vi "MEMR-Initialize SGDA.vi"(0 "Data folder":path, 5 "Params":T32, 11 "error in (no error)":errorcluster) -> (4 "AO":T2 {"noiseChan"."Filter"."Stages"."IIR Filter"."Forward Coefficients" format="%.4f"; "noiseChan"."Filter"."Stages"."IIR Filter"."Reverse Coefficients" format="%.4f"}, 12 "Step In":T1, 14 "Step Out":T1, 15 "error out":errorcluster)   [LabVIEW 2020]
uses:
  Typedefs/MEMR-Params.ctl
  Typedefs/MEMR-Probe.ctl
  Typedefs/MEMR-Elicitor.ctl
  Human Studies/SFM Frontend/LV Source/Typedefs/HSTS-Transducer.ctl
  Typedefs/MEMR-Sequence.ctl
  Typedefs/MEMR-Analysis.ctl
  Typedefs/MEMR-Timing.ctl
  Typedefs/MEMR-AO Data.ctl
  Signal Synthesis VIs/3rd Generation/XControls/Stimulus Channel (G3)/Full Stimulus Channel Data.ctl
  Signal Synthesis VIs/3rd Generation/XControls/Waveform XControls/Waveform (G3)/Waveform Data.ctl
  Signal Synthesis VIs/3rd Generation/Waveform VIs/Waveform Enum (V3).ctl
  Signal Synthesis VIs/3rd Generation/XControls/Waveform XControls/Tone (G3)/Tone.Properties.ctl
  Signal Synthesis VIs/Waveform VIs/Pulse Train VIs/Pulse Train Params.ctl
  Signal Synthesis VIs/Waveform VIs/Pulse Train VIs/Pulse Polarity.ctl
  Signal Synthesis VIs/Waveform VIs/Pulse Train VIs/PT-Continuous State.ctl
  Signal Synthesis VIs/3rd Generation/Waveform VIs/Noise VIs/Noise (G3).ctl
  Signal Synthesis VIs/3rd Generation/Waveform VIs/Noise VIs/Noise (G3).Properties.ctl
  Signal Synthesis VIs/3rd Generation/Waveform VIs/Noise VIs/Noise (G3).Data.ctl
  Signal Synthesis VIs/Waveform VIs/File VIs/StimFile-Params.ctl
  Signal Synthesis VIs/Waveform VIs/FM Sweep VIs/FM Sweep Params.ctl
  Signal Synthesis VIs/Waveform VIs/Chirp Train VIs/Chirp Train.ctl
  Signal Synthesis VIs/Waveform VIs/Chirp Train VIs/Chirp Train Params.ctl
  Signal Synthesis VIs/Waveform VIs/Complex Tone VIs/CT-Params.ctl
  Signal Synthesis VIs/Waveform VIs/Complex Tone VIs/CT-Phase Enum.ctl
  Signal Synthesis VIs/Waveform VIs/Complex Tone VIs/CT-Runtime Data.ctl
  Signal Synthesis VIs/3rd Generation/XControls/Waveform XControls/FM Tone/Data.ctl
  Signal Synthesis VIs/3rd Generation/XControls/Waveform XControls/Vowel/Vowel.Properties.ctl
  Signal Synthesis VIs/3rd Generation/Waveform VIs/Ramp VIs/Ramp.Properties.ctl
  Signal Synthesis VIs/3rd Generation/XControls/Filter (G3)/Filter Data.ctl
  Signal Synthesis VIs/3rd Generation/XControls/Filter (G3)/Filter Type.ctl
  Signal Synthesis VIs/Filter VIs/Filter-Bandwidth Units.ctl
  Signal Synthesis VIs/Controls/Burst XCtl/Burst Data.ctl
  Signal Synthesis VIs/3rd Generation/XControls/Level (G3)/Level Data.ctl
  Signal Synthesis VIs/3rd Generation/XControls/Level (G3)/Level Units (G3).ctl
  Signal Synthesis VIs/3rd Generation/XControls/Advanced Options (G3)/Advanced Options (G3).ctl
  Signal Synthesis VIs/Modulation VIs/SAM VIs/SAM Params.ctl
  Signal Synthesis VIs/3rd Generation/Typedefs/Destination.ctl
  Typedefs/MEMR-Sequence Step.ctl
  Signal Synthesis VIs/3rd Generation/XControls/Filter (G3)/Filter (G3).xctl
  Signal Synthesis VIs/3rd Generation/XControls/Level (G3)/Level (G3).xctl
  Signal Synthesis VIs/Controls/Burst XCtl/Burst Control.xctl
  Signal Synthesis VIs/3rd Generation/XControls/Waveform XControls/Tone (G3)/Tone (G3).xctl
  Signal Synthesis VIs/3rd Generation/XControls/Waveform XControls/FM Tone/FM Tone.xctl
  Signal Synthesis VIs/3rd Generation/XControls/Waveform XControls/Vowel/Vowel.xctl
  Signal Synthesis VIs/3rd Generation/XControls/Waveform XControls/Waveform (G3)/Waveform (G3).xctl
  Signal Synthesis VIs/3rd Generation/XControls/Advanced Options (G3)/Advanced Options (G3).xctl
  Signal Synthesis VIs/3rd Generation/XControls/Stimulus Channel (G3)/Stimulus Channel (G3).xctl
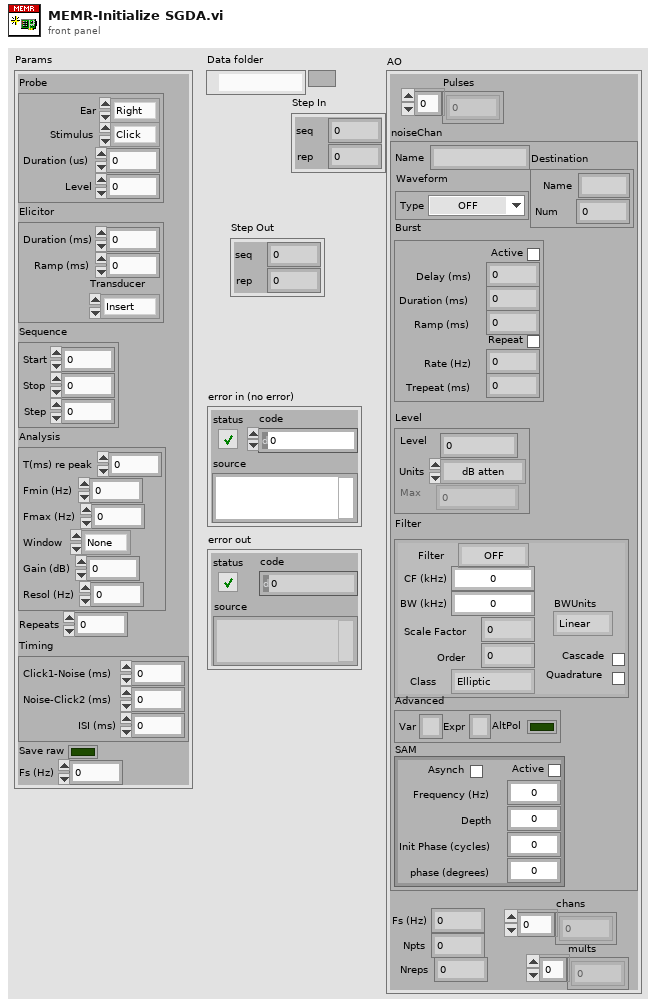
[diagram p1: front panel]
types:
  T1 = typedef "MEMR-Sequence Step.ctl" = cluster{"seq":i32, "rep":i32}
  T2 = typedef "MEMR-AO Data.ctl" = cluster{"Pulses":dbl[], "noiseChan":T3, "Fs (Hz)":dbl, "Npts":i32, "mults":dbl[], "chans":i32[], "Nreps":i32}
  T3 = typedef "Stimulus Channel (G3).xctl/Full Stimulus Channel Data.ctl" = cluster{"Waveform":T4, "Filter":T23, "Burst":T26, "Level":T27, "Name":string, "Advanced":T29, "SAM":T30, "Destination":T31}
  T4 = typedef "Waveform (G3).xctl/Waveform Data.ctl" = cluster{"Type":T5, "Tone":T6, "Pulse Train":T7, "Noise":T10, "File":T13, "FMSweep":T14, "Chirp Train":T15, "Complex Tone":cluster{"Params":T17, "Data":T19}, "FM":T20, "Vowel":T21, "Ramp":T22}
  T5 = typedef "Waveform Enum (V3).ctl" = enum16{"OFF", "Tone", "Noise", "Pulse Train", "File", "FM Sweep", "Chirp Train", "Complex Tone", "FM Tone", "Vowel", "Ramp"}
  T6 = typedef "Tone (G3).xctl/Tone.Properties.ctl" = cluster{"Frequency (kHz)":dbl, "Phase (cycles)":dbl, "Random phase":bool}
  T7 = typedef "Pulse Train Params.ctl" = cluster{"Pulse width (us)":dbl, "Pulse rate (Hz)":dbl, "Gap (ms)":dbl, "Polarity":T8, "PT State":T9, "Asynch":bool}
  T8 = typedef "Pulse Polarity.ctl" = enum16{"POS", "NEG", "POS-NEG", "NEG-POS"}
  T9 = typedef "PT-Continuous State.ctl" = cluster{"Template":dbl[], "Nperiod":i32, "Index":i32, "Pulse Rate (Hz)":dbl, "Phase (cycles)":dbl, "Noff":i32}
  T10 = typedef "Noise (G3).ctl" = cluster{"Properties":T11, "Data":T12}
  T11 = typedef "Noise (G3).Properties.ctl" = cluster{"InvFilt":bool, "Aweight":bool, "Seed":i32, "Tokens":i32, "Brickwall":bool}
  T12 = typedef "Noise (G3).Data.ctl" = cluster{"TokenNum":i32}
  T13 = typedef "StimFile-Params.ctl" = cluster{"Filename":path, "Signal":dbl[], "Channel":i32, "stream":bool, "offset":i32, "nreps":i32, "loops":i32, "Randomize":bool, "order":i32[], "Seed":i32, "Tokens":i32}
  T14 = typedef "FM Sweep Params.ctl" = cluster{"Rate (oct/s)":dbl, "Fmin (Hz)":dbl, "Fmax (Hz)":dbl, "Ramp (ms)":dbl, "Linear":bool}
  T15 = typedef "Chirp Train.ctl" = cluster{"Params":T16, "Data":cluster{"WF":dbl[]}}
  T16 = typedef "Chirp Train Params.ctl" = cluster{"Fmin (kHz)":dbl, "Fmax (kHz)":dbl, "Compensate":bool, "Duration (ms)":dbl}
  T17 = typedef "CT-Params.ctl" = cluster{"F0 (Hz)":dbl, "Band":cluster{"Flow (Hz)":dbl, "Fhigh (Hz)":dbl}, "Phase":T18, "Min F0 (Hz)":dbl, "Max F0 (Hz)":dbl, "ContinRandPhase":bool, "Max peak factor":dbl, "Max mod depth":dbl, "MinHarmNum":i32, "MaxHarmNum":i32, "Level Mode":enum16{"per component", "overall rms"}, "% jitter":dbl}
  T18 = typedef "CT-Phase Enum.ctl" = enum16{"Cosine", "Random", "Alternating"}
  T19 = typedef "CT-Runtime Data.ctl" = cluster{"Ncomp":i32, "MinHarm":i32, "Phase":dbl[], "Amplitude":dbl[], "Npts/frame":i32, "Last F0":dbl, "Fmin":dbl, "Fmax":dbl, "Lslope":dbl, "randphase":bool, "overall rms":bool, "fmult":dbl[], "jittered":bool}
  T20 = typedef "FM Tone.xctl/Data.ctl" = cluster{"Carrier (kHz)":dbl, "ModRate (Hz)":dbl, "Depth (Hz)":dbl, "Phase (cycles)":dbl}
  T21 = typedef "Vowel.xctl/Vowel.Properties.ctl" = cluster{"Freqs":string, "Set level":enum16{"Total", "Per component"}, "Freq":dbl[], "weights":dbl[]}
  T22 = typedef "Ramp.Properties.ctl" = cluster{"Duration (ms)":dbl}
  T23 = typedef "Filter (G3).xctl/Filter Data.ctl" = cluster{"Type":T24, "CF (kHz)":dbl, "BW (kHz)":dbl, "Cascade":bool, "Quadrature":bool, "Scale Factor":dbl, "Stages":cluster{"IIR Filter":cluster{"filter structure":enum32{"IIR 2nd Order", "IIR 4th Order"}, "Reverse Coefficients":dbl[], "Forward Coefficients":dbl[]}, "State":dbl[]}[], "Class":enum16{"Elliptic", "Butterworth"}, "Order":i32, "BWUnits":T25}
  T24 = typedef "Filter (G3).xctl/Filter Type.ctl" = enum16{"OFF", "Lowpass", "Highpass", "Bandpass", "Bandstop"}
  T25 = typedef "Filter-Bandwidth Units.ctl" = enum16{"Linear", "Octaves", "Min-Max"}
  T26 = typedef "Burst Control.xctl/Burst Data.ctl" = cluster{"Active":bool, "Delay (ms)":dbl, "Duration (ms)":dbl, "Ramp (ms)":dbl, "Rate (Hz)":dbl, "Trepeat (ms)":dbl, "Repeat":bool}
  T27 = typedef "Level (G3).xctl/Level Data.ctl" = cluster{"Level":dbl, "Units":T28, "Max":dbl, "Data":cluster{"Multiplier":dbl, "Cal File":path, "Cal":cluster{"Freq (Hz)":dbl[], "Mag (dB SPL)":dbl[], "Phase (deg)":dbl[]}, "audiogram":path}}
  T28 = typedef "Level (G3).xctl/Level Units (G3).ctl" = enum16{"dB atten", "dB SPL", "dB re 1 Vrms", "dB V/Hz½", "mW", "dB HL", "Volts", "dB mW"}
  T29 = typedef "Advanced Options (G3).xctl/Advanced Options (G3).ctl" = cluster{"AltPol":bool, "Var":string, "Expr":string}
  T30 = typedef "SAM Params.ctl" = cluster{"Active":bool, "Frequency (Hz)":dbl, "Depth":dbl, "Init Phase (cycles)":dbl, "phase (degrees)":dbl, "Asynch":bool}
  T31 = typedef "Destination.ctl" = cluster{"Name":string, "Num":i32}
  T32 = typedef "MEMR-Params.ctl" = cluster{"Probe":T33, "Elicitor":T34, "Sequence":T36, "Analysis":T37, "Repeats":i32, "Timing":T38, "Save raw":bool, "Fs (Hz)":dbl}
  T33 = typedef "MEMR-Probe.ctl" = cluster{"Ear":enum16{"Right", "Left"}, "Stimulus":enum16{"Click", "Chirp"}, "Duration (us)":dbl, "Level":dbl}
  T34 = typedef "MEMR-Elicitor.ctl" = cluster{"Duration (ms)":dbl, "Ramp (ms)":dbl, "Transducer":T35}
  T35 = typedef "HSTS-Transducer.ctl" = enum16{"Insert", "TDH-39", "HD300", "ER-10X"}
  T36 = typedef "MEMR-Sequence.ctl" = cluster{"Start":dbl, "Stop":dbl, "Step":dbl}
  T37 = typedef "MEMR-Analysis.ctl" = cluster{"T(ms) re peak":dbl, "Fmin (Hz)":dbl, "Fmax (Hz)":dbl, "Window":enum16{"None", "Hanning", "Hamming"}, "Gain (dB)":dbl, "Resol (Hz)":dbl}
  T38 = typedef "MEMR-Timing.ctl" = cluster{"Click1-Noise (ms)":dbl, "Noise-Click2 (ms)":dbl, "ISI (ms)":dbl}
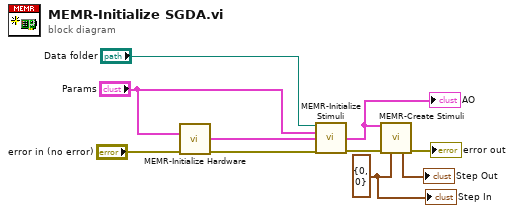
[diagram p0: block diagram]
diagram:
  w2 = T1 {"seq"=0, "rep"=0} ("Step In")
  n1 = call "MEMR-Initialize Hardware.vi"("Params"="Params", "error in (no error)"="error in (no error)") -> ("AO"=w8:T2, "error out"=w7:errorcluster)  [unwired: 12 in]
  n2 = call "MEMR-Initialize Stimuli.vi"("Data folder"="Data folder", "Params"="Params", "AO in"=w8, "error in (no error)"=w7) -> ("AO out"=w3:T2, "error out"=w5:errorcluster)  [unwired: 10 in]
  "AO" <- w3
  n3 = call "MEMR-Create Stimuli.vi"("AO"=w3, "error in (no error)"=w5, "Step In"=w2) -> ("Step Out"=→"Step Out":T1, "error out"=→"error out":errorcluster)  [unwired: 10 in, 1 out]
  "Step In" <- w2
